vi "StoreAllCtrlsConfig.vi"(11 "VI in":refnum<vi>) -> ()   [LabVIEW 2020]
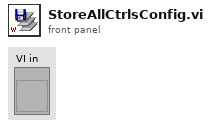
[diagram p1: front panel]
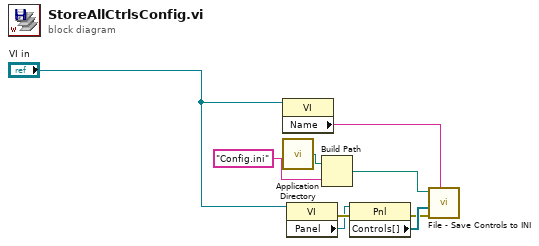
[diagram p0: block diagram]
diagram:
  n1 = property class="VI"(reference="VI in") -> ("Name"=w9:string)  [unwired: 1 in, 2 out]
  n2 = call <vilib>:"Application Directory.vi"() -> ("Application Directory"=w7:path)
  n3 = property class="VI"(reference="VI in") -> (error out=w4:errorcluster, "Panel"=w3:refnum<vi>)  [unwired: 1 in, 1 out]
  n4 = Build Path(base path=w7, name or relative path="Config.ini") -> (appended path=w2:path)
  n5 = property class="Pnl"(reference=w3, error in=w4) -> (error out=w5:errorcluster, "Controls[]"=w6:refnum<vi>[])  [unwired: 1 out]
  n6 = call "File - Save Controls to INI.vi"("Section"=w9, "error in (no error)"=w5, "Array of References"=w6, "INI File"=w2) -> ()  [unwired: 7 in, 1 out]
